vi "lockincore_nn.vi"(0 "Lock-in parameters":T2={"frequency"=2282.0, "order"=3, "low cutoff freq: fl"=200.0} {"low cutoff freq: fl" format="%#_13g"; "frequency" format="%0.2p"}, 1 "start/stop":bool=TRUE, 5 "sampling info":cluster{"Fs":dbl, "#s":dbl}={"Fs"=200000.0, "#s"=100000.0} {"Fs" format="%.2p"}, 7 "signal task in":refnum<k21>, 9 "Reference Phase (degrees)":dbl, 11 "error in (no error)":errorcluster) -> (3 "output cluster":T1, 4 "lock-in output":cluster{"R":dbl, "Theta":dbl, "X":dbl, "Y":dbl}, 6 "task out":refnum<k21>, 8 "photodiode":waveform(dbl), 10 "reference out":waveform(dbl), 14 "ref 90":waveform(dbl), 15 "error out":errorcluster)   [LabVIEW 2015]
uses:
  <vilib>/Analysis/3filter.llb/Filter Passband Type.ctl
  <vilib>/DAQmx/read.llb/DAQmx Read (Analog Wfm 1Chan NSamp).vi
  <vilib>/Analysis/baseanly.llb/Mean (DBL).vi
  <vilib>/DAQmx/miscellaneous.llb/DAQmx Fill In Error Info.vi
  <vilib>/Analysis/3filter.llb/Butterworth Filter (DBL).vi
  <vilib>/Analysis/NI_AALBase.lvlib
panel:
  # "Locks into frequency to find modulation amplitude"
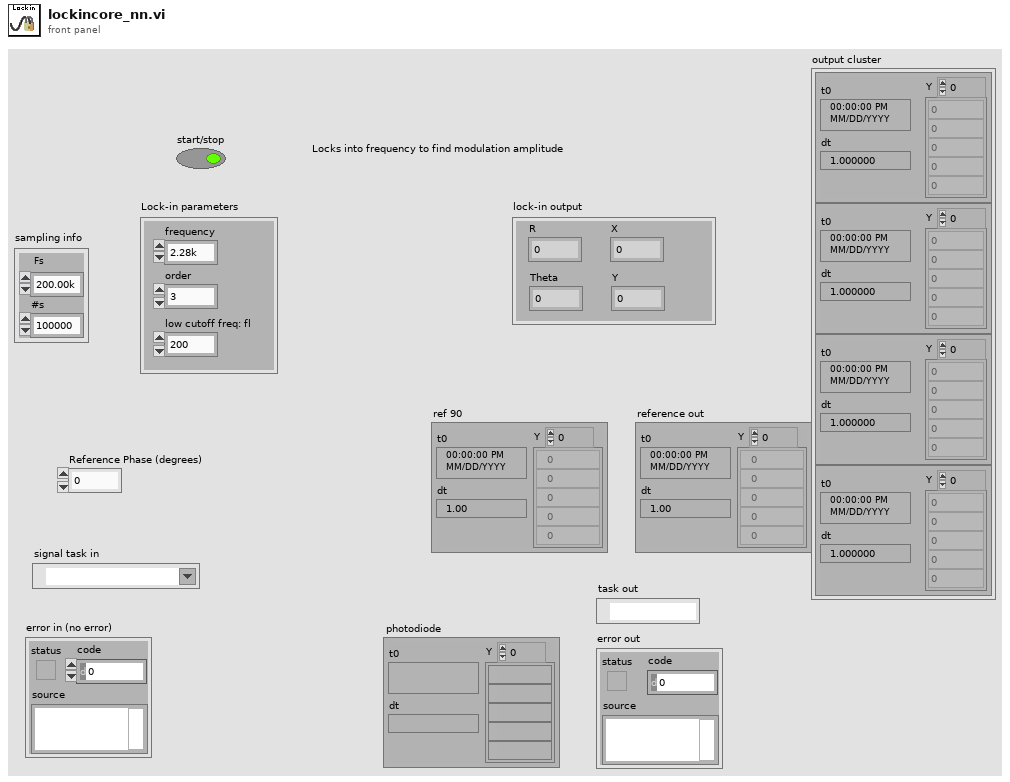
[diagram p1: front panel]
types:
  T1 = cluster{"Waveform":waveform(dbl), "Waveform":waveform(dbl), "Waveform":waveform(dbl), "Waveform":waveform(dbl)}
  T2 = cluster{"frequency":dbl, "order":i32, "low cutoff freq: fl":dbl}
  T3 = typedef "NI_AALBase.lvlib/Filter Passband Type.ctl" = enum32{"Lowpass", "Highpass", "Bandpass", "Bandstop"}
  T4 = cluster{"mean":dbl, "mean":dbl, "mean":dbl, "mean":dbl}
  T5 = cluster{waveform(dbl), waveform(dbl), waveform(dbl), waveform(dbl)}
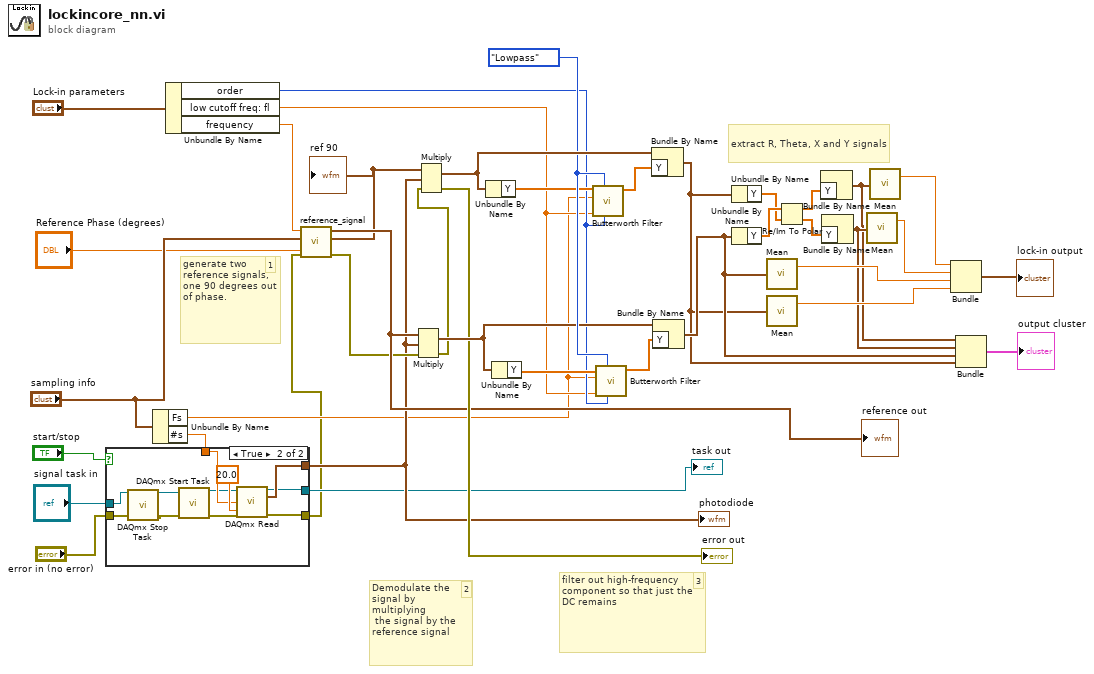
[diagram p0: block diagram]
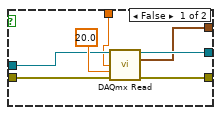
[diagram p2: hidden frame]
diagram:
  w37 = Filter_Passband_Type."Lowpass" ("filter type")
  # "1"
  # "2"
  # "3"
  # "extract R, Theta, X and Y signals"
  # "filter out high-frequency component so that just the DC remains"
  # "Demodulate the signal by multiplying\n the signal by the reference signal"
  # "generate two reference signals, one 90 degrees out of phase."
  n1 = Unbundle By Name("sampling info") -> ("Fs"=w12:dbl, "#s"=w13:dbl)
  n2 = case shown="True" "start/stop" {
    tunnel: [w42 w57] -> w15
    tunnel: w13 -> [w41 w56]
    tunnel: [w46 w52] -> w5
    tunnel: "signal task in" -> [w45 w51]
    tunnel: "error in (no error)" -> [w44 w48]
    tunnel: [w43 w53] -> w2
    frame False {
      n3 = call-poly <vilib>:"DAQmx Read.vi"("task/channels in"=w45, "number of samples per channel"=w41, "timeout"=20.0, "error in"=w44) -> ("task out"=w46:refnum<k21>, "data"=w42:waveform(dbl), "error out"=w43:errorcluster)  [unwired: 9 in]
    }
    frame True {
      n4 = call <vilib>:"DAQmx Stop Task.vi"("task/channels in"=w51, "error in"=w48) -> ("task out"=w50:refnum<k21>, "error out"=w49:errorcluster)  [unwired: 12 in]
      n5 = call <vilib>:"DAQmx Start Task.vi"("task/channels in"=w50, "error in"=w49) -> ("task out"=w55:refnum<k21>, "error out"=w54:errorcluster)  [unwired: 12 in]
      n6 = call-poly <vilib>:"DAQmx Read.vi"("task/channels in"=w55, "number of samples per channel"=w56, "timeout"=20.0, "error in"=w54) -> ("task out"=w52:refnum<k21>, "data"=w57:waveform(dbl), "error out"=w53:errorcluster)  [unwired: 9 in]
    }
  }
  "task out" <- w5
  "photodiode" <- w15
  n7 = Unbundle By Name("Lock-in parameters") -> ("order"=w32:i32, "low cutoff freq: fl"=w31:dbl, "frequency"=w20:dbl)
  n8 = call "reference_signal.vi"("error in (no error)"=w2, "Phase (degrees)"="Reference Phase (degrees)", "sampling info"="sampling info", "frequency"=w20) -> ("error out"=w18:errorcluster, "ref 90"=w16:waveform(dbl), "ref"=w19:waveform(dbl))  [unwired: 5 in]
  "reference out" <- w19
  "ref 90" <- w16
  n9 = Multiply(1:w15, 2:w19, 4:w18) -> (0:w34:waveform(dbl), 3:w17:errorcluster)
  n10 = Multiply(1:w15, 2:w16, 4:w17) -> (0:w38:waveform(dbl), 3:→"error out":errorcluster)
  n11 = Unbundle By Name(w38) -> ("Y"=w36:dbl[])
  n12 = Unbundle By Name(w34) -> ("Y"=w40:dbl[])
  n13 = call-poly <vilib>:"Butterworth Filter.vi"("order"=w32, "filter type"=w37, "low cutoff freq: fl"=w31, "sampling freq: fs"=w12, "X"=w36) -> ("Filtered X"=w39:dbl[])  [unwired: 3 in, 1 out]
  n14 = call-poly <vilib>:"Butterworth Filter.vi"("order"=w32, "filter type"=w37, "low cutoff freq: fl"=w31, "sampling freq: fs"=w12, "X"=w40) -> ("Filtered X"=w35:dbl[])  [unwired: 3 in, 1 out]
  n15 = Bundle By Name(cluster=w38, "Y"=w39) -> (w7:waveform(dbl))
  n16 = Bundle By Name(cluster=w34, "Y"=w35) -> (w8:waveform(dbl))
  n17 = Unbundle By Name(w7) -> ("Y"=w28:dbl[])
  n18 = Unbundle By Name(w8) -> ("Y"=w29:dbl[])
  n19 = call-poly <vilib>:"Mean.vi"("X"=w8) -> ("mean"=w22:dbl)  [unwired: 1 out]
  n20 = call-poly <vilib>:"Mean.vi"("X"=w7) -> ("mean"=w21:dbl)  [unwired: 1 out]
  n21 = Re/Im To Polar(2:w28, 3:w29) -> (0:w26:dbl[], 1:w27:dbl[])
  n22 = Bundle By Name("Y"=w27) -> (w10:waveform(dbl))  [unwired: 1 in]
  n23 = Bundle By Name("Y"=w26) -> (w11:waveform(dbl))  [unwired: 1 in]
  n24 = call-poly <vilib>:"Mean.vi"("X"=w11) -> ("mean"=w23:dbl)  [unwired: 1 out]
  n25 = call-poly <vilib>:"Mean.vi"("X"=w10) -> ("mean"=w24:dbl)  [unwired: 1 out]
  n26 = Bundle("mean"=w24, "mean"=w23, "mean"=w22, "mean"=w21) -> (→"lock-in output":T4)  [unwired: 1 in]
  n27 = Bundle(w10, w11, w8, w7) -> (→"output cluster":T5)  [unwired: 1 in]
